vi "VisionExecute.v.vi"   [LabVIEW 2023]
uses:
  <vilib>/Rock Robotics/WPI/ThirdParty/PhotonPoseStrategy_ENUM.ctl
  <vilib>/Rock Robotics/WPI/ThirdParty/JAS_Junk/TrajLib/TypeDef/POSE2D.ctl
  <vilib>/Rock Robotics/WPI/ThirdParty/JAS_Junk/TrajLib/TypeDef/TRANSLATION2D.ctl
  <vilib>/Rock Robotics/WPI/ThirdParty/JAS_Junk/TrajLib/TypeDef/ROTATION2D.ctl
  <vilib>/Rock Robotics/WPI/ThirdParty/JAS_Junk/TrajLib/VI/Util_GetTime_U32.vi
  <vilib>/Rock Robotics/WPI/ThirdParty/PhotonVisionLib/SubVI/PhotonPipelineResult_Unpack.vi
  <vilib>/Rock Robotics/WPI/ThirdParty/PhotonVisionLib/SubVI/PhotonPipelineResult_SetTimeStampSecs.vi
  <vilib>/Rock Robotics/WPI/ThirdParty/PhotonVisionLib/SubVI/PhotonPipelineResult_GetLatency_Millis.vi
  <vilib>/Rock Robotics/WPI/ThirdParty/PhotonVisionLib/SubVI/PhotonPipelineResult_GetTimeStampSecs.vi
  <vilib>/Rock Robotics/WPI/ThirdParty/JAS_Junk/TrajLib/VI/Transform3d_Equals.vi
  <vilib>/Rock Robotics/WPI/ThirdParty/PhotonVisionLib/SubVI/PhotonPoseEstimator_SetCamera.vi
  <vilib>/Rock Robotics/WPI/ThirdParty/PhotonVisionLib/SubVI/PhotonPoseEstimator_SetPrimaryStategy.vi
  <vilib>/Rock Robotics/WPI/ThirdParty/PhotonVisionLib/SubVI/PhotonPoseEstimator_SetMultiTagFallbackStrategy.vi
  <vilib>/Rock Robotics/WPI/ThirdParty/PhotonVisionLib/SubVI/PhotonPoseEstimator_SetHighestAmbiguity.vi
  <vilib>/Rock Robotics/WPI/ThirdParty/PhotonVisionLib/SubVI/PhotonPoseEstimator_SetRobotToCameraTransform.vi
  <vilib>/Rock Robotics/WPI/ThirdParty/PhotonVisionLib/SubVI/PhotonPoseEstimator_New.vi
  <vilib>/Rock Robotics/WPI/ThirdParty/JAS_Junk/TrajLib/VI/AprilTagFieldLayout_NewSelect.vi
  <vilib>/Rock Robotics/WPI/ThirdParty/PhotonVisionLib/SubVI/PhotonPoseEstimator_SetLastPose.vi
  <vilib>/Rock Robotics/WPI/ThirdParty/PhotonVisionLib/SubVI/PhotonPoseEstimator_Update_PipeResult.vi
  <vilib>/Rock Robotics/WPI/ThirdParty/PhotonVisionLib/SubVI/PhotonPoseEstimator_SetReferencePose.vi
  <vilib>/Rock Robotics/WPI/ThirdParty/PhotonVisionLib/SubVI/PhotonEstimatedRobotPose_GetAll.vi
  <vilib>/Rock Robotics/WPI/ThirdParty/JAS_Junk/TrajLib/VI/Pose3d_ToPose2d.vi
  <vilib>/Rock Robotics/WPI/ThirdParty/JAS_Junk/TrajLib/VI/Quaternion_New.vi
  <vilib>/Rock Robotics/WPI/ThirdParty/JAS_Junk/TrajLib/Conv_Deg_Radians.vi
  <vilib>/Rock Robotics/WPI/ThirdParty/JAS_Junk/TrajLib/Translation2d_GetDistance.vi
  <vilib>/Rock Robotics/WPI/ThirdParty/JAS_Junk/TrajLib/Rotation2d_Minus.vi
  <vilib>/Rock Robotics/WPI/ThirdParty/JAS_Junk/TrajLib/Rotation2d_GetRadians.vi
  <vilib>/Rock Robotics/WPI/ThirdParty/JAS_Junk/TrajLib/Translation2d_Equals.vi
  <vilib>/Rock Robotics/WPI/ThirdParty/JAS_Junk/TrajLib/Rotation2d_Equals.vi
  <vilib>/Rock Robotics/WPI/ThirdParty/PhotonVisionLib/SubVI/Packet_decode_Flt64.vi
  <vilib>/Rock Robotics/WPI/ThirdParty/PhotonVisionLib/SubVI/Packet_decode_ByteI8.vi
  <vilib>/Rock Robotics/WPI/ThirdParty/PhotonVisionLib/SubVI/PhotonTrackedTarget_Unpack.vi
  <vilib>/Rock Robotics/WPI/ThirdParty/PhotonVisionLib/SubVI/PhotonMultiTargetPNPResult_unpack.vi
  <vilib>/Rock Robotics/WPI/ThirdParty/PhotonVisionLib/SubVI/PhotonPipelineResult_New.vi
  <vilib>/Rock Robotics/WPI/ThirdParty/JAS_Junk/TrajLib/VI/Transform3d_GetTranslation3d.vi
  <vilib>/Rock Robotics/WPI/ThirdParty/JAS_Junk/TrajLib/VI/Transform3d_GetRotation3d.vi
  <vilib>/Rock Robotics/WPI/ThirdParty/JAS_Junk/TrajLib/VI/Rotation3d_Equals.vi
  <vilib>/Rock Robotics/WPI/ThirdParty/JAS_Junk/TrajLib/VI/Translation3d_Equals.vi
  <vilib>/Rock Robotics/WPI/ThirdParty/PhotonVisionLib/SubVI/PhotonTargetModel_New_AprilTag16h5.vi
  <vilib>/Rock Robotics/WPI/ThirdParty/JAS_Junk/TrajLib/VI/AprilTagFieldLayout_New2022.vi
  <vilib>/Rock Robotics/WPI/ThirdParty/JAS_Junk/TrajLib/VI/AprilTagFieldLayout_New2023.vi
  <vilib>/Rock Robotics/WPI/ThirdParty/JAS_Junk/TrajLib/VI/AprilTagFieldLayout_New2024.vi
  <vilib>/Rock Robotics/WPI/ThirdParty/PhotonVisionLib/SubVI/PhotonPoseEstimator_Update_All.vi
  <vilib>/Rock Robotics/WPI/ThirdParty/JAS_Junk/TrajLib/VI/Pose3d_getTranslation3d.vi
  <vilib>/Rock Robotics/WPI/ThirdParty/JAS_Junk/TrajLib/VI/Pose3d_getRotation3d.vi
  <vilib>/Rock Robotics/WPI/ThirdParty/JAS_Junk/TrajLib/VI/Translation3d_ToTranslation2d.vi
  <vilib>/Rock Robotics/WPI/ThirdParty/JAS_Junk/TrajLib/VI/Rotation3d_ToRotation2d.vi
  <vilib>/Rock Robotics/WPI/ThirdParty/JAS_Junk/TrajLib/Pose2d_New_TRRO.vi
  <vilib>/Rock Robotics/WPI/ThirdParty/JAS_Junk/TrajLib/Util_CalcDist.vi
  <vilib>/Rock Robotics/WPI/ThirdParty/JAS_Junk/TrajLib/Rotation2d_UnaryMinus.vi
  <vilib>/Rock Robotics/WPI/ThirdParty/JAS_Junk/TrajLib/Rotation2d_RotateBy.vi
  <vilib>/Rock Robotics/WPI/ThirdParty/PhotonVisionLib/SubVI/TargetCorner_New.vi
  <vilib>/Rock Robotics/WPI/ThirdParty/PhotonVisionLib/SubVI/Packet_decode_Int32.vi
  <vilib>/Rock Robotics/WPI/ThirdParty/PhotonVisionLib/SubVI/Packet_decode_Transform3d.vi
  <vilib>/Rock Robotics/WPI/ThirdParty/PhotonVisionLib/SubVI/PhotonPNPResult_unpackt.vi
  <vilib>/Rock Robotics/WPI/ThirdParty/PhotonVisionLib/SubVI/PhotonMultiTargetPNPResult_New.vi
  <vilib>/Rock Robotics/WPI/ThirdParty/PhotonVisionLib/SubVI/PhotonMultiTargetPNPResult_MAX_IDS.vi
  <vilib>/Rock Robotics/WPI/ThirdParty/PhotonVisionLib/SubVI/Packet_decode_Int16.vi
  <vilib>/Rock Robotics/WPI/ThirdParty/JAS_Junk/TrajLib/VI/Rotation3d_GetQuaterion.vi
  <vilib>/Rock Robotics/WPI/ThirdParty/JAS_Junk/TrajLib/VI/Quaternion_Equals.vi
  <vilib>/Rock Robotics/WPI/ThirdParty/PhotonVisionLib/SubVI/PhotonTargetModel_New_RectPlanar.vi
  <vilib>/Rock Robotics/WPI/ThirdParty/JAS_Junk/TrajLib/VI/AprilTagFieldLayout_New.vi
  <vilib>/Rock Robotics/WPI/ThirdParty/JAS_Junk/TrajLib/VI/Pose3d_New_Trans3dRot3d.vi
  <vilib>/Rock Robotics/WPI/ThirdParty/JAS_Junk/TrajLib/VI/Rotation3d_Create_Quaternion.vi
  <vilib>/Rock Robotics/WPI/ThirdParty/JAS_Junk/TrajLib/VI/AprilTag_New.vi
  <vilib>/Rock Robotics/WPI/ThirdParty/PhotonVisionLib/SubVI/PhotonPoseEstimator_GetEmptyPose.vi
  <vilib>/Rock Robotics/WPI/ThirdParty/PhotonVisionLib/SubVI/PhotonPoseEstimator_lowestAmbiguityStrategy.vi
  <vilib>/Rock Robotics/WPI/ThirdParty/PhotonVisionLib/SubVI/PhotonPoseEstimator_closestToCameraHeightStrategy.vi
  <vilib>/Rock Robotics/WPI/ThirdParty/PhotonVisionLib/SubVI/PhotonPoseEstimator_closestToReferencePoseStrategy.vi
  <vilib>/Rock Robotics/WPI/ThirdParty/PhotonVisionLib/SubVI/PhotonPoseEstimator_GetReferencePose.vi
  <vilib>/Rock Robotics/WPI/ThirdParty/PhotonVisionLib/SubVI/PhotonPoseEstimator_GetLastPose.vi
  <vilib>/Rock Robotics/WPI/ThirdParty/PhotonVisionLib/SubVI/PhotonPoseEstimator_averageBestTargetsStrategy.vi
  <vilib>/Rock Robotics/WPI/ThirdParty/PhotonVisionLib/SubVI/PhotonPoseEstimator_multiTagOnCoprocStrategy.vi
  <vilib>/Rock Robotics/WPI/ThirdParty/JAS_Junk/TrajLib/Translation2d_Create.vi
  <vilib>/Rock Robotics/WPI/ThirdParty/JAS_Junk/TrajLib/Rotation2d_CreateAngle.vi
  <vilib>/Rock Robotics/WPI/ThirdParty/JAS_Junk/TrajLib/VI/Rotation3d_GetXYZ.vi
  <vilib>/Rock Robotics/WPI/ThirdParty/JAS_Junk/TrajLib/Rotation2d_CreateXY.vi
  <vilib>/Rock Robotics/WPI/ThirdParty/PhotonVisionLib/SubVI/Packet_decode_Boolean.vi
  <vilib>/Rock Robotics/WPI/ThirdParty/PhotonVisionLib/SubVI/PhotonPNPResult_New_Empty.vi
  <vilib>/Rock Robotics/WPI/ThirdParty/PhotonVisionLib/SubVI/PhotonPNPResult_New.vi
  <vilib>/Rock Robotics/WPI/ThirdParty/JAS_Junk/TrajLib/VI/Quaternion_Get_Vect.vi
  <vilib>/Rock Robotics/WPI/ThirdParty/JAS_Junk/TrajLib/VI/Quaternion_Get_W.vi
  <vilib>/Rock Robotics/WPI/ThirdParty/PhotonVisionLib/SubVI/PhotonTargetModel_New.vi
  <vilib>/Rock Robotics/WPI/ThirdParty/JAS_Junk/TrajLib/VI/AprilTag_GetAll.vi
  <vilib>/Rock Robotics/WPI/ThirdParty/JAS_Junk/TrajLib/VI/Quaternion_Normalize.vi
  <vilib>/Rock Robotics/WPI/ThirdParty/JAS_Junk/TrajLib/VI/Rotation3d_Create_AxisAngle.vi
  <vilib>/Rock Robotics/WPI/ThirdParty/JAS_Junk/TrajLib/VI/Pose3d_New.vi
  <vilib>/Rock Robotics/WPI/ThirdParty/PhotonVisionLib/SubVI/PhotonPipelineResult_HasTargets.vi
  <vilib>/Rock Robotics/WPI/ThirdParty/PhotonVisionLib/SubVI/PhotonPipelineResult_GetTargets.vi
  <vilib>/Rock Robotics/WPI/ThirdParty/PhotonVisionLib/SubVI/PhotonTrackedTarget_GetPoseAmbiguity.vi
  <vilib>/Rock Robotics/WPI/ThirdParty/PhotonVisionLib/SubVI/PhotonTrackedTarget_GetFiducialId.vi
  <vilib>/Rock Robotics/WPI/ThirdParty/PhotonVisionLib/SubVI/PhotonPoseEstimator_GetFieldTags.vi
  <vilib>/Rock Robotics/WPI/ThirdParty/JAS_Junk/TrajLib/VI/AprilTagFieldLayout_GetTagPose.vi
  <vilib>/Rock Robotics/WPI/ThirdParty/JAS_Junk/TrajLib/VI/Pose3d_TransformBy.vi
  <vilib>/Rock Robotics/WPI/ThirdParty/PhotonVisionLib/SubVI/PhotonTrackedTarget_GetBestCameraToTarget.vi
  <vilib>/Rock Robotics/WPI/ThirdParty/JAS_Junk/TrajLib/VI/Transform3d_Inverse.vi
  <vilib>/Rock Robotics/WPI/ThirdParty/PhotonVisionLib/SubVI/PhotonPoseEstimator_GetRobotToCameraTransform.vi
  <vilib>/Rock Robotics/WPI/ThirdParty/PhotonVisionLib/SubVI/PhotonPoseEstimator_GetHighestAmbiguity.vi
  <vilib>/Rock Robotics/WPI/ThirdParty/PhotonVisionLib/SubVI/PhotonEstimatedRobotPose_New.vi
  <vilib>/Rock Robotics/WPI/ThirdParty/PhotonVisionLib/SubVI/PhotonPoseEstimator_closestToCameraHeightStrategy_calc.vi
  <vilib>/Rock Robotics/WPI/ThirdParty/PhotonVisionLib/SubVI/PhotonTrackedTarget_GetAltCameraToTarget.vi
  <vilib>/Rock Robotics/WPI/ThirdParty/PhotonVisionLib/SubVI/PhotonPoseEstimator_closestToReferencePoseStrategy_calc.vi
  <vilib>/Rock Robotics/WPI/ThirdParty/PhotonVisionLib/SubVI/PhotonPoseEstimator_averageBestTargetsStrategy_calc.vi
  <vilib>/Rock Robotics/WPI/ThirdParty/JAS_Junk/TrajLib/VI/Rotation3d_Plus.vi
  <vilib>/Rock Robotics/WPI/ThirdParty/JAS_Junk/TrajLib/VI/Translation3d_Plus.vi
  <vilib>/Rock Robotics/WPI/ThirdParty/JAS_Junk/TrajLib/VI/Translation3d_Times.vi
  <vilib>/Rock Robotics/WPI/ThirdParty/JAS_Junk/TrajLib/VI/Rotation3d_Times.vi
  <vilib>/Rock Robotics/WPI/ThirdParty/JAS_Junk/TrajLib/VI/Rotation3d_Create_Default.vi
  <vilib>/Rock Robotics/WPI/ThirdParty/JAS_Junk/TrajLib/VI/Translation3d_Create_Default.vi
  <vilib>/Rock Robotics/WPI/ThirdParty/JAS_Junk/TrajLib/VI/Pose3d_New_Default.vi
  <vilib>/Rock Robotics/WPI/ThirdParty/JAS_Junk/TrajLib/VI/Pose3d_Plus.vi
  <vilib>/Rock Robotics/WPI/ThirdParty/JAS_Junk/TrajLib/VI/Pose3d_RelativeTo.vi
  <vilib>/Rock Robotics/WPI/ThirdParty/JAS_Junk/TrajLib/VI/AprilTagFieldLayout_GetOriginPosition.vi
  <vilib>/Rock Robotics/WPI/ThirdParty/PhotonVisionLib/SubVI/PhotonPipelineResult_GetMultiTagResult.vi
  <vilib>/Rock Robotics/WPI/ThirdParty/JAS_Junk/TrajLib/VI/Quaternion_Get_All.vi
  <vilib>/Rock Robotics/WPI/ThirdParty/JAS_Junk/TrajLib/VI/Quaternion_New_Default.vi
  <vilib>/Rock Robotics/WPI/ThirdParty/JAS_Junk/TrajLib/VI/Vector_Norm.vi
  <vilib>/Rock Robotics/WPI/ThirdParty/JAS_Junk/TrajLib/VecBuilder_ArrayBy1Fill.vi
  <vilib>/Rock Robotics/WPI/ThirdParty/JAS_Junk/TrajLib/VI/Translation3d_RotateBy.vi
  <vilib>/Rock Robotics/WPI/ThirdParty/JAS_Junk/TrajLib/Transform2d_Create_TransRot.vi
  <vilib>/Rock Robotics/WPI/ThirdParty/JAS_Junk/TrajLib/VI/Rotation3d_UnaryMinus.vi
  <vilib>/Rock Robotics/WPI/ThirdParty/JAS_Junk/TrajLib/VI/Translation3d_UnaryMinus.vi
  <vilib>/Rock Robotics/WPI/ThirdParty/JAS_Junk/TrajLib/VI/Transform3d_GetXYZ.vi
  <vilib>/Rock Robotics/WPI/ThirdParty/JAS_Junk/TrajLib/VI/Pose3d_getXYZ.vi
  <vilib>/Rock Robotics/WPI/ThirdParty/PhotonVisionLib/SubVI/PhotonPoseEstimator_CalcDifference.vi
  <vilib>/Rock Robotics/WPI/ThirdParty/JAS_Junk/TrajLib/VI/Rotation3d_RotateBy.vi
  <vilib>/Rock Robotics/WPI/ThirdParty/JAS_Junk/TrajLib/VI/Translation3d_GetXYZ.vi
  <vilib>/Rock Robotics/WPI/ThirdParty/JAS_Junk/TrajLib/VI/Transform3d_Create_Pose3dPose3d.vi
  <vilib>/Rock Robotics/WPI/ThirdParty/JAS_Junk/TrajLib/MatBuilder_Create.vi
  <vilib>/Rock Robotics/WPI/ThirdParty/JAS_Junk/TrajLib/VI/Quaternion_Times.vi
  <vilib>/Rock Robotics/WPI/ThirdParty/JAS_Junk/TrajLib/VI/Quaternion_Inverse.vi
  <vilib>/Rock Robotics/WPI/ThirdParty/JAS_Junk/TrajLib/VI/Translation3d_GetDistance.vi
  <vilib>/Rock Robotics/WPI/ThirdParty/JAS_Junk/TrajLib/VI/Translation3d_Minus.vi
  <vilib>/Rock Robotics/WPI/ThirdParty/JAS_Junk/TrajLib/VI/Rotation3d_Minus.vi
  <vilib>/Rock Robotics/SystemInterfaces/Utilities/FPGA_UtilitiesRead LocalTime.vi
  <vilib>/Rock Robotics/WPI/ThirdParty/JAS_Junk/TrajLib/VI/Util_GetTime_U64.vi
  <vilib>/Rock Robotics/Network Tables/NT Write Number.vi
  VisionGlobal.vi
  <vilib>/Rock Robotics/Network Tables/NT Read Value.vi
  <vilib>/Rock Robotics/Network Tables/NT Read Raw.vi
  <vilib>/Rock Robotics/WPI/ThirdParty/JAS_Junk/TrajLib/Trajectory_Library.lvlib
  <vilib>/Rock Robotics/WPI/ThirdParty/PhotonVisionLib/PhotonVisionLib.lvlib
types:
  T1 = typedef "PhotonVisionLib.lvlib/PhotonPoseStrategy_ENUM.ctl" = enum16{"LOWEST_AMBIGUITY", "CLOSEST_TO_CAMERA_HEIGHT", "CLOSEST_TO_REFERENCE_POSE", "CLOSEST_TO_LAST_POSE", "AVERAGE_BEST_TARGETS", "MULTI_TAG_PNP_ON_COPROCESSOR", "MULTI_TAG_PNP_ON_RIO"}
  T2 = enum16{"2022 Rapid React", "2023 Charged Up", "2024 Crescendo"}
  T3 = typedef "Trajectory_Library.lvlib/TRANSLATION3D.ctl" = cluster{"X":dbl, "Y":dbl, "Z":dbl}
  T4 = typedef "Trajectory_Library.lvlib/ROTATION3D.ctl" = cluster{"Q_quaternion":T5}
  T5 = typedef "Trajectory_Library.lvlib/QUATERNION.ctl" = cluster{"R":dbl, "V":dbl[]}
  T6 = typedef "Trajectory_Library.lvlib/TRANSFORM3D.ctl" = cluster{"TRANSLATION3D":T3, "ROTATION3D":T4, "XF":bool}
  T7 = typedef "PhotonVisionLib.lvlib/PhotonPipelineResultType.ctl" = cluster{"TargetCount":i32, "Latency_MilliSec":dbl, "Targets":T8[], "TimeStampSec":dbl, "PhotonMultiTargetPNPResult":T10}
  T8 = typedef "PhotonVisionLib.lvlib/PhotonTrackedTargetType.ctl" = cluster{"Yaw":dbl, "Pitch":dbl, "Area":dbl, "Skew":dbl, "MinAreaRectCorners":T9[], "BestCameraToTarget":T6, "FiiducialId":i32, "AltCameraToTarget":T6, "PoseAmbiguity":dbl, "DetectedCorners":T9[]}
  T9 = typedef "PhotonVisionLib.lvlib/TargetCornerType.ctl" = cluster{"X":dbl, "Y":dbl}
  T10 = typedef "PhotonVisionLib.lvlib/PhotonMultiTargetPNPResultType.ctl" = cluster{"PhotonPNPResult":T11, "FiducialIDsUsed":i16[]}
  T11 = typedef "PhotonVisionLib.lvlib/PhotonPNPResultType.ctl" = cluster{"IsPresent":bool, "bestReprojErr":dbl, "altReprojErr":dbl, "ambiguity":dbl, "Best":T6, "Alt":T6}
  T12 = typedef "Trajectory_Library.lvlib/POSE2D.ctl" = cluster{"TRANSLATION":T13, "ROTATION":T14}
  T13 = typedef "Trajectory_Library.lvlib/TRANSLATION2D.ctl" = cluster{"X":dbl, "Y":dbl}
  T14 = typedef "Trajectory_Library.lvlib/ROTATION2D.ctl" = cluster{"VALUE":dbl, "COS":dbl, "SIN":dbl}
  T15 = typedef "PhotonVisionLib.lvlib/PhotonPoseEstimator_Configuration.ctl" = cluster{"Primary Strategy":T1, "Camera":string, "Initial Pose":T16, "HighestAmbiguity":dbl, "Use Custom Field":bool, "Custom AprilTag Field":T17, "RobotToCamera":T6, "FallBack Strategy":T1, "BaseNTName":string, "AprilTagField":enum16{"2022 Rapid React", "2023 Charged Up", "2024 Crescendo"}}
  T16 = typedef "Trajectory_Library.lvlib/POSE3D.ctl" = cluster{"Translation3d":T3, "Rotation3d":T4}
  T17 = typedef "Trajectory_Library.lvlib/AprilTagFieldLayout.ctl" = cluster{"AprilTagMap":map{i32, T18}, "FieldLength":dbl, "FieldWidth":dbl, "OriginPosition ":T19, "OriginPose3d":T16}
  T18 = typedef "Trajectory_Library.lvlib/AprilTag.ctl" = cluster{"ID":i32, "POSE3D":T16}
  T19 = typedef "Trajectory_Library.lvlib/AprilTagFieldLayoutOrignPosition_ENUM.ctl" = enum16{"kBlueAllianceWallRightSide,", "kRedAllianceWallRightSide,"}
  T20 = typedef "Trajectory_Library.lvlib/SWERVE_DRIVE_KINEMATICS.ctl" = cluster{"NumModules":i32, "InverseKinematics":T21, "ForwardKinematics":T21, "Modules":T13[], "PrevCoR":T13, "SavedModuleStates":T22[]}
  T21 = typedef "NI_Matrix.lvlib/RealMatrix.ctl" = dbl[][]
  T22 = typedef "Trajectory_Library.lvlib/SWERVE_DRIVE_MODULE_STATE.ctl" = cluster{"Speed":dbl, "Angle":T14}
  T23 = typedef "Trajectory_Library.lvlib/SWERVE_DRIVE_MODULE_POSITION.ctl" = cluster{"Distance":dbl, "Angle":T14, "P":bool}
  T24 = typedef "Trajectory_Library.lvlib/SWERVE_DRIVE_POSE_EST2_CONFIG.ctl" = cluster{"Wheel_Locations M":T13[], "Odom X std dev M":dbl, "Odom Y std dev M":dbl, "Odom Heading std dev Rad":dbl, "Vision X std dev M":dbl, "Vision Y std dev M":dbl, "Vision Heading std dev Rad":dbl}
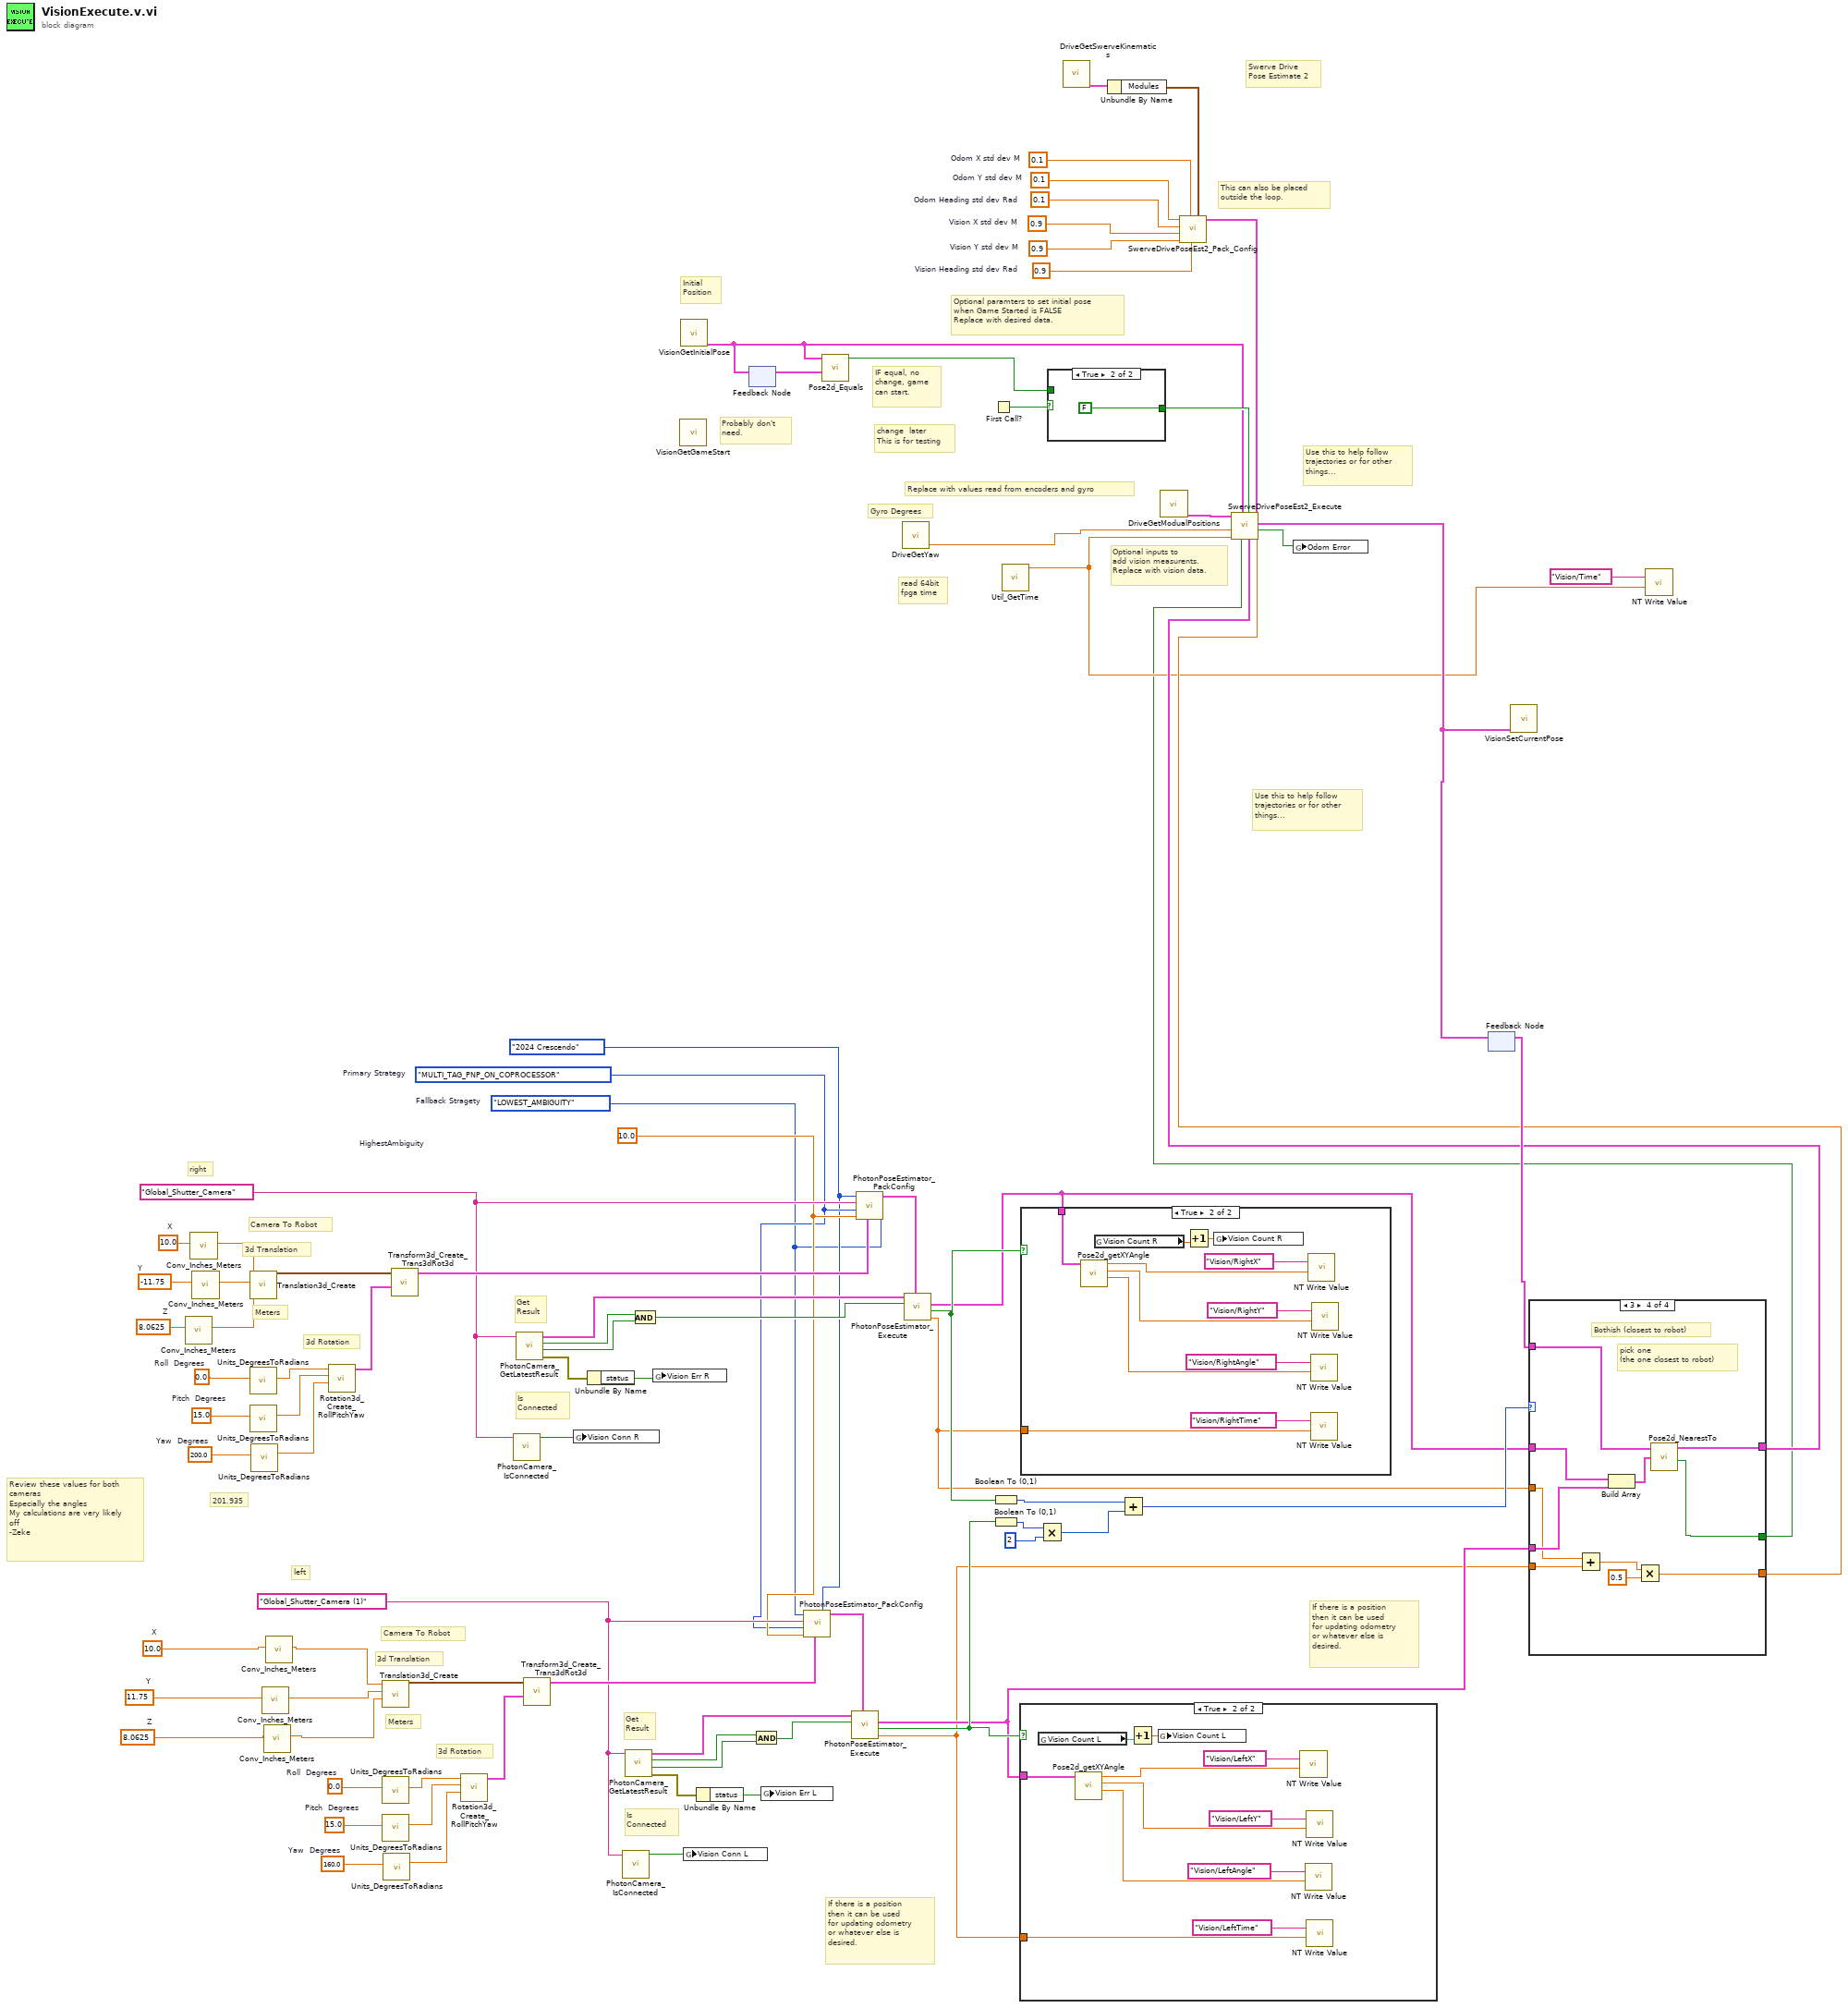
[diagram p0: block diagram]
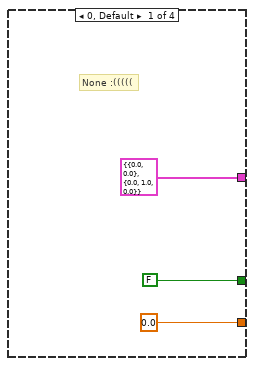
[diagram p3: hidden frame]
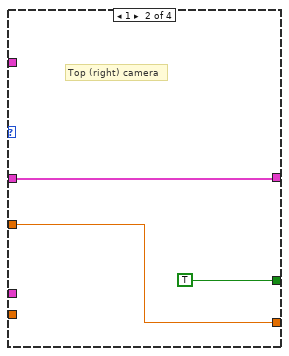
[diagram p4: hidden frame]
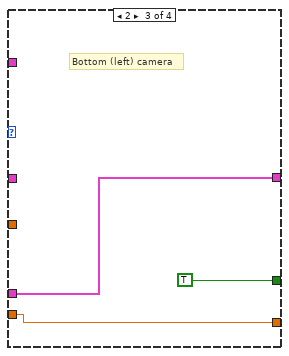
[diagram p5: hidden frame]
diagram:
  w13 = PhotonPoseStrategy_ENUM."LOWEST_AMBIGUITY"  # Fallback Stragety
  w14 = T2."2024 Crescendo" ("AprilTagField")
  w24 = 0.1  # Odom Y std dev M
  w25 = 0.1  # Odom Heading std dev Rad
  w26 = 0.9  # Vision X std dev M
  w27 = 0.9  # Vision Y std dev M
  w28 = 0.1  # Odom X std dev M
  w29 = 0.9  # Vision Heading std dev Rad
  w62 = 0.0  # Roll  Degrees
  w61 = 15.0  # Pitch  Degrees
  w60 = 160.0  # Yaw  Degrees
  w47 = 8.0625  # Z
  w51 = 10.0  # X
  w49 = 11.75  # Y
  w56 = "Global_Shutter_Camera (1)" ("CameraName")
  w80 = 0.0  # Roll  Degrees
  w79 = 15.0  # Pitch  Degrees
  w78 = 200.0  # Yaw  Degrees
  w41 = 8.0625  # Z
  w45 = 10.0  # X
  w43 = -11.75  # Y
  w39 = 10.0  # HighestAmbiguity
  w38 = PhotonPoseStrategy_ENUM."MULTI_TAG_PNP_ON_COPROCESSOR"  # Primary Strategy
  w74 = "Global_Shutter_Camera" ("CameraName")
  # "Probably don't\nneed."
  # "IF equal, no \nchange, game\ncan start."
  # "Initial\nPosition"
  # "201.935"
  # "change  later\nThis is for testing"
  # "Review these values for both cameras\nEspecially the angles\nMy calculations are very likely off\n-Zeke"
  # "Optional inputs to\nadd vision measurents.\nReplace with vision data."
  # "Replace with values read from encoders and gyro"
  # "Optional paramters to set initial pose\nwhen Game Started is FALSE\nReplace with desired data."
  # "read 64bit\nfpga time"
  # "This can also be placed \noutside the loop."
  # "Use this to help follow\ntrajectories or for other\nthings..."
  # "Swerve Drive \nPose Estimate 2"
  # "Use this to help follow\ntrajectories or for other\nthings..."
  # "right"
  # "left"
  # "If there is a position\nthen it can be used\nfor updating odometry\nor whatever else is \ndesired."
  # "Meters"
  # "Camera To Robot"
  # "3d Rotation"
  # "3d Translation"
  # "Is\nConnected"
  # "Get\nResult"
  # "If there is a position\nthen it can be used\nfor updating odometry\nor whatever else is \ndesired."
  # "Meters"
  # "Camera To Robot"
  # "3d Rotation"
  # "3d Translation"
  # "Is\nConnected"
  # "Get\nResult"
  # "Gyro Degrees"
  n1 = call <vilib>:"Conv_Inches_Meters.vi"("INCH"=w41) -> ("Meters"=w40:dbl)  [unwired: 10 in]
  n2 = call <vilib>:"Conv_Inches_Meters.vi"("INCH"=w45) -> ("Meters"=w44:dbl)  [unwired: 10 in]
  n3 = call <vilib>:"Conv_Inches_Meters.vi"("INCH"=w43) -> ("Meters"=w42:dbl)  [unwired: 10 in]
  n4 = call <vilib>:"Translation3d_Create.vi"("Z"=w40, "Y"=w42, "X"=w44) -> ("TRANSLATION3D"=w81:T3)  [unwired: 8 in]
  n5 = call <vilib>:"Units_DegreesToRadians.vi"("Degrees"=w80) -> ("Radians"=w77:dbl)  [unwired: 10 in]
  n6 = call <vilib>:"Units_DegreesToRadians.vi"("Degrees"=w79) -> ("Radians"=w76:dbl)  [unwired: 10 in]
  n7 = call <vilib>:"Units_DegreesToRadians.vi"("Degrees"=w78) -> ("Radians"=w75:dbl)  [unwired: 10 in]
  n8 = call <vilib>:"Conv_Inches_Meters.vi"("INCH"=w49) -> ("Meters"=w48:dbl)  [unwired: 10 in]
  n9 = call <vilib>:"Conv_Inches_Meters.vi"("INCH"=w47) -> ("Meters"=w46:dbl)  [unwired: 10 in]
  n10 = call <vilib>:"Conv_Inches_Meters.vi"("INCH"=w51) -> ("Meters"=w50:dbl)  [unwired: 10 in]
  n11 = call <vilib>:"Rotation3d_Create_RollPitchYaw.vi"("Yaw"=w75, "Pitch"=w76, "Roll"=w77) -> ("Rotation3d"=w82:T4)  [unwired: 8 in]
  n12 = call <vilib>:"Translation3d_Create.vi"("Z"=w46, "Y"=w48, "X"=w50) -> ("TRANSLATION3D"=w63:T3)  [unwired: 8 in]
  n13 = call <vilib>:"Units_DegreesToRadians.vi"("Degrees"=w62) -> ("Radians"=w59:dbl)  [unwired: 10 in]
  n14 = call <vilib>:"Units_DegreesToRadians.vi"("Degrees"=w61) -> ("Radians"=w58:dbl)  [unwired: 10 in]
  n15 = call <vilib>:"Units_DegreesToRadians.vi"("Degrees"=w60) -> ("Radians"=w57:dbl)  [unwired: 10 in]
  n16 = call <vilib>:"Transform3d_Create_Trans3dRot3d.vi"("Rotation3d"=w82, "Translation3d"=w81) -> ("Transform3d"=w83:T6)  [unwired: 9 in]
  n17 = call <vilib>:"Rotation3d_Create_RollPitchYaw.vi"("Yaw"=w57, "Pitch"=w58, "Roll"=w59) -> ("Rotation3d"=w64:T4)  [unwired: 8 in]
  n18 = call <vilib>:"PhotonCamera_IsConnected.vi"("CameraName"=w74) -> ("IsConnected"=w72:bool)  [unwired: 9 in, 1 out]
  n19 = call <vilib>:"PhotonCamera_GetLatestResult.vi"("CameraName"=w74) -> ("error out"=w71:errorcluster, "New Data"=w87:bool, "HasTargets"=w86:bool, "PipelineResult"=w84:T7)  [unwired: 7 in]
  n20 = call <vilib>:"Transform3d_Create_Trans3dRot3d.vi"("Rotation3d"=w64, "Translation3d"=w63) -> ("Transform3d"=w65:T6)  [unwired: 9 in]
  n21 = global write "VisionGlobal.vi" "Vision Conn R"(w72) -> ()
  n22 = Unbundle By Name(w71) -> ("status"=w70:bool)
  n23 = call <vilib>:"PhotonCamera_IsConnected.vi"("CameraName"=w56) -> ("IsConnected"=w54:bool)  [unwired: 9 in, 1 out]
  n24 = call <vilib>:"PhotonCamera_GetLatestResult.vi"("CameraName"=w56) -> ("error out"=w53:errorcluster, "New Data"=w69:bool, "HasTargets"=w68:bool, "PipelineResult"=w66:T7)  [unwired: 7 in]
  n25 = And(x=w86, y=w87) -> (x .and. y?=w85:bool)
  n26 = global write "VisionGlobal.vi" "Vision Err R"(w70) -> ()
  n27 = call "VisionGetGameStart.vi"() -> ()  [unwired: 11 in, 1 out]
  n28 = call "VisionGetInitialPose.vi"() -> ("InitialPose"=w3:T12)  [unwired: 10 in]
  n29 = global write "VisionGlobal.vi" "Vision Conn L"(w54) -> ()
  n30 = Unbundle By Name(w53) -> ("status"=w52:bool)
  n31 = feedback-in #1(w3) -> ()
  n32 = feedback #1() -> (w2:T12)  [unwired: 1 in]
  n33 = And(x=w68, y=w69) -> (x .and. y?=w67:bool)
  n34 = global write "VisionGlobal.vi" "Vision Err L"(w52) -> ()
  n35 = call <vilib>:"PhotonPoseEstimator_PackConfig.vi"("FallBack Strategy"=w13, "RobotToCamera"=w65, "HighestAmbiguity"=w39, "PirmaryStrategy"=w38, "Camera"=w56, "AprilTagField"=w14) -> ("PoseEstimator_Configuration"=w55:T15)  [unwired: 5 in]
  n36 = call <vilib>:"Pose2d_Equals.vi"("other POSE"=w2, "in POSE"=w3) -> ("Equals"=w1:bool)  [unwired: 9 in]
  n37 = call <vilib>:"PhotonPoseEstimator_Execute.vi"("Configuration"=w55, "PIpeline Has \nNew Results"=w67, "PipelineResult"=w66) -> ("TimeStamp_Seconds"=w8:dbl, "New Pose Found"=w36:bool, "EstimatedPose2d"=w10:T12)  [unwired: 2 in, 4 out]
  n38 = call <vilib>:"PhotonPoseEstimator_PackConfig.vi"("FallBack Strategy"=w13, "RobotToCamera"=w83, "HighestAmbiguity"=w39, "PirmaryStrategy"=w38, "Camera"=w74, "AprilTagField"=w14) -> ("PoseEstimator_Configuration"=w73:T15)  [unwired: 5 in]
  n39 = call "DriveGetYaw.vi"() -> ("Yaw"=w19:dbl)  [unwired: 11 in]
  n40 = call <vilib>:"PhotonPoseEstimator_Execute.vi"("Configuration"=w73, "PIpeline Has \nNew Results"=w85, "PipelineResult"=w84) -> ("TimeStamp_Seconds"=w7:dbl, "New Pose Found"=w37:bool, "EstimatedPose2d"=w9:T12)  [unwired: 2 in, 4 out]
  n41 = First Call?() -> (First Call?: T/F=w11:bool)
  n42 = Boolean To (0,1)(Boolean=w37) -> (0, 1=w32:i16)
  n43 = Boolean To (0,1)(Boolean=w36) -> (0, 1=w35:i16)
  n44 = call <vilib>:"Util_GetTime.vi"() -> ("FPGA_Time_Seconds"=w5:dbl)  [unwired: 9 in, 2 out]
  n45 = case shown="True" w36 {
    tunnel: w10 -> [_ w95]
    tunnel: w8 -> [_ w88]
    frame False {
    }
    frame True {
      n46 = global read "VisionGlobal.vi" "Vision Count L"() -> (w97:dbl)
      n47 = call <vilib>:"Pose2d_getXYAngle.vi"("in POSE"=w95) -> ("Angle"=w90:dbl, "Y"=w91:dbl, "X"=w92:dbl)  [unwired: 8 in]
      n48 = Increment(x=w97) -> (x+1=w98:dbl)
      n49 = global write "VisionGlobal.vi" "Vision Count L"(w98) -> ()
      n50 = call-poly <vilib>:"NT Write Value.vi"("value"=w92, "name"="Vision/LeftX") -> ()  [unwired: 9 in, 1 out]
      n51 = call-poly <vilib>:"NT Write Value.vi"("value"=w90, "name"="Vision/LeftAngle") -> ()  [unwired: 9 in, 1 out]
      n52 = call-poly <vilib>:"NT Write Value.vi"("value"=w91, "name"="Vision/LeftY") -> ()  [unwired: 9 in, 1 out]
      n53 = call-poly <vilib>:"NT Write Value.vi"("value"=w88, "name"="Vision/LeftTime") -> ()  [unwired: 9 in, 1 out]
    }
  }
  n54 = case shown="True" w37 {
    tunnel: w9 -> [_ w101]
    tunnel: w7 -> [_ w99]
    frame False {
    }
    frame True {
      n55 = call <vilib>:"Pose2d_getXYAngle.vi"("in POSE"=w101) -> ("Angle"=w102:dbl, "Y"=w103:dbl, "X"=w104:dbl)  [unwired: 8 in]
      n56 = global read "VisionGlobal.vi" "Vision Count R"() -> (w108:dbl)
      n57 = Increment(x=w108) -> (x+1=w109:dbl)
      n58 = global write "VisionGlobal.vi" "Vision Count R"(w109) -> ()
      n59 = call-poly <vilib>:"NT Write Value.vi"("value"=w104, "name"="Vision/RightX") -> ()  [unwired: 9 in, 1 out]
      n60 = call-poly <vilib>:"NT Write Value.vi"("value"=w102, "name"="Vision/RightAngle") -> ()  [unwired: 9 in, 1 out]
      n61 = call-poly <vilib>:"NT Write Value.vi"("value"=w99, "name"="Vision/RightTime") -> ()  [unwired: 9 in, 1 out]
      n62 = call-poly <vilib>:"NT Write Value.vi"("value"=w103, "name"="Vision/RightY") -> ()  [unwired: 9 in, 1 out]
    }
  }
  n63 = Multiply(x=w35, y=i16 2) -> (x*y=w33:i16)
  n64 = case shown="True" w11 {
    tunnel: [w110 FALSE] -> w12
    tunnel: w1 -> [w110 _]
    frame False {
    }
    frame True {
    }
  }
  n65 = call "DriveGetSwerveKinematics.vi"() -> ("SWERVE_DRIVE_KINEMATICS"=w16:T20)  [unwired: 11 in]
  n66 = Unbundle By Name(w16) -> ("Modules"=w15:T13[])
  n67 = Add(x=w32, y=w33) -> (x+y=w31:i16)
  n68 = call "DriveGetModualPositions.vi"() -> ("Swerve_Drive_Modual_Positions"=w20:T23[])  [unwired: 11 in]
  n69 = call <vilib>:"SwerveDrivePoseEst2_Pack_Config.vi"("Wheel_Locations M"=w15, "Vision Heading std dev Rad"=w29, "Odom X std dev M"=w28, "Vision Y std dev M"=w27, "Vision X std dev M"=w26, "Odom Heading std dev Rad"=w25, "Odom Y std dev M"=w24) -> ("SwervePoseEst2Config"=w23:T24)  [unwired: 4 in]
  n70 = feedback #2() -> (w30:T12)  [unwired: 1 in]
  n71 = case shown="3" w31 {
    tunnel: w9 -> [_ w116 _ w129]
    tunnel: w10 -> [_ _ w119 w128]
    tunnel: w30 -> [_ _ _ w130]
    tunnel: [FALSE ("Found") TRUE ("Found") TRUE ("Found") w126] -> w4
    tunnel: w7 -> [_ w117 _ w125]
    tunnel: w8 -> [_ _ w120 w124]
    tunnel: [T12 {"TRANSLATION"={"X"=0.0, "Y"=0.0}, "ROTATION"={"VALUE"=0.0, "COS"=1.0, "SIN"=0.0}} ("Nearest Pose") w116 w119 w127] -> w18
    tunnel: [0.0 w117 w120 w121] -> w17
    frame 0, Default {
      # "None :((((("
    }
    frame 1 {
      # "Top (right) camera"
    }
    frame 2 {
      # "Bottom (left) camera"
    }
    frame 3 {
      # "pick one \n(the one closest to robot)"
      # "Bothish (closest to robot)"
      n72 = Add(x=w125, y=w124) -> (x+y=w123:dbl)
      n73 = Build Array(w129, w128) -> (w131:T12[])
      n74 = Multiply(x=w123, y=0.5) -> (x*y=w121:dbl)
      n75 = call <vilib>:"Pose2d_NearestTo.vi"("other POSE"=w131, "in POSE"=w130) -> ("Found"=w126:bool, "Nearest Pose"=w127:T12)  [unwired: 8 in]
    }
  }
  n76 = call <vilib>:"SwerveDrivePoseEst2_Execute.vi"("Vision TImeStamp_Seconds"=w17, "SwervePoseEst2Config"=w23, "visionRobotPose"=w18, "Game Started"=w12, "Add Vision Meas"=w4, "InitialPose"=w3, "Pass Through Time"=w5, "Gyro Degrees"=w19, "Module Positions"=w20) -> ("Error"=w21:bool, "Estimated Pose"=w22:T12)  [unwired: 1 in]
  n77 = global write "VisionGlobal.vi" "Odom Error"(w21) -> ()
  n78 = feedback-in #2(w22) -> ()
  n79 = call "VisionSetCurrentPose.vi"("Current Pose"=w22) -> ()  [unwired: 11 in]
  n80 = call-poly <vilib>:"NT Write Value.vi"("value"=w5, "name"="Vision/Time") -> ()  [unwired: 9 in, 1 out]
